vi "ReadSpec校准.vi"() -> (3 "补偿值":T3={"甩线补偿值"={"下边"=23.0, "距离上边"=10.0, "左边"=7.2, "右边"=25.8}, "补偿甩线坐标偏移"={"X"=40.0, "Y"=70.0}, "mark点补偿"={"X"=-48.38, "Y"=-84.85}, "出线补偿值"=25.8, "mark规格"={"X下限"=-48.38, "X上限"=-84.85, "Y下限"=0.0, "Y 上限"=0.0, "angle下限"=0.0, "angle上限"=0.0}} {"mark规格"."angle上限" format="%#.3f"; "mark规格"."angle下限" format="%#.3f"; "mark规格"."Y下限" format="%#.3f"; "mark规格"."X下限" format="%#.3f"; "mark点补偿"."X" format="%#.3f"; "补偿甩线坐标偏移"."X" format="%#.3f"})   [LabVIEW 2014]
uses:
  Controls/XYPos.ctl
  Global.vi
  <vilib>/Utility/file.llb/Read From Spreadsheet File (string).vi
panel:
  out "all rows":string[][](array[string]) caption="所有行"
  out "数组":dbl[](array[numeric])
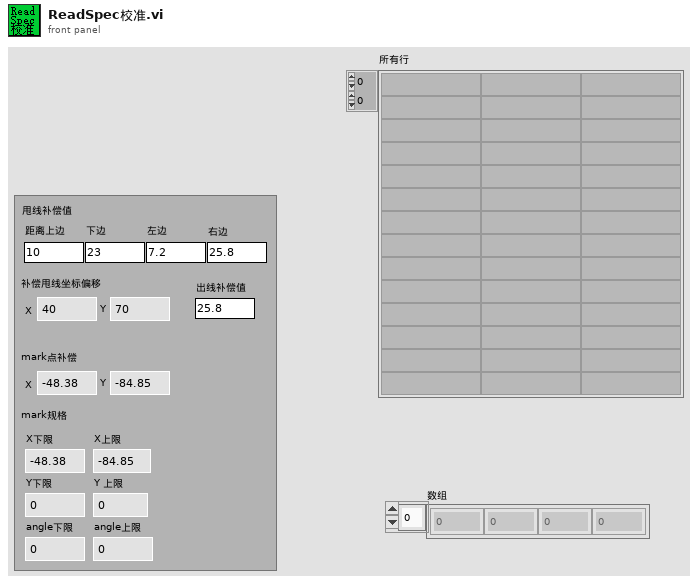
[diagram p1: front panel]
types:
  T1 = typedef "XYPos.ctl" = cluster{"X":dbl, "Y":dbl}
  T2 = typedef "mark规格.ctl" = cluster{"X下限":dbl, "X上限":dbl, "Y下限":dbl, "Y 上限":dbl, "angle下限":dbl, "angle上限":dbl}
  T3 = cluster{"甩线补偿值":cluster{"下边":dbl, "距离上边":dbl, "左边":dbl, "右边":dbl}, "补偿甩线坐标偏移":T1, "mark点补偿":T1, "出线补偿值":dbl, "mark规格":T2}
  T4 = cluster{"[0]":dbl, "[1]":dbl, "[2]":dbl, "[3]":dbl}
  T5 = cluster{"[0]":dbl, "[1]":dbl, "[2]":dbl, "[3]":dbl, "[4]":dbl, "[5]":dbl}
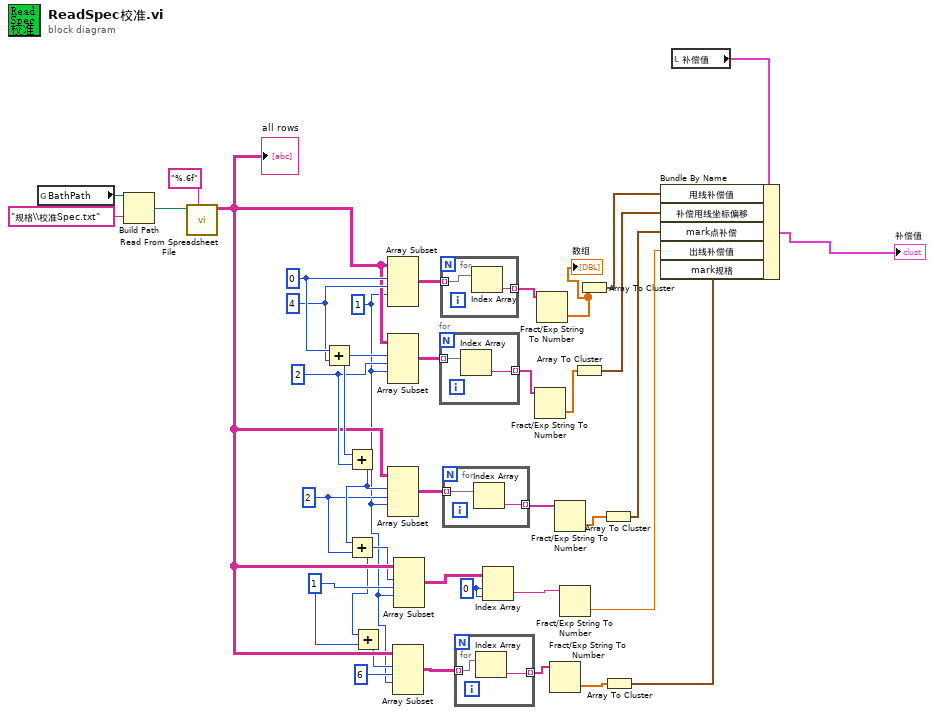
[diagram p0: block diagram]
diagram:
  w11 = 0 ("索引 (行)")
  w9 = 1 ("长度")
  w23 = 2 ("长度")
  w26 = 4
  w18 = 2 ("长度")
  w27 = 0 ("索引")
  w5 = 1 ("索引")
  n1 = global read "Global.vi" "BathPath"() -> (w37:path)
  n2 = Build Path(base path=w37, name or relative path="规格\\校准Spec.txt" ("名称或相对路径")) -> (appended path=w31:path)
  n3 = call-poly <vilib>:"Read From Spreadsheet File.vi"("format (%s)"="%.6f" ("format (%.3f)"), "file path (dialog if empty)"=w31) -> ("all rows"=w10:string[][])  [unwired: 5 in, 4 out]
  "all rows" <- w10
  n4 = Add(x=w27, y=w26) -> (x+y=w24:i32)
  n5 = Add(x=w24, y=w23) -> (x+y=w19:i32)
  n6 = Add(x=w19, y=w18) -> (x+y=w8:i32)
  n7 = Add(x=w8, y=w9) -> (x+y=w7:i32)
  n8 = Array Subset ("数组子集")(array=w10, index (row)=w27, length (row)=w26, index (col)=w5) -> (w35:string[][])  [unwired: 1 in]
  n9 = Array Subset ("数组子集")(array=w10, index (row)=w24, length (row)=w23, index (col)=w5) -> (w33:string[][])  [unwired: 1 in]
  n10 = Array Subset ("数组子集")(array=w10, index (row)=w19, length (row)=w18, index (col)=w5) -> (w30:string[][])  [unwired: 1 in]
  n11 = Array Subset ("数组子集")(array=w10, index (row)=w7, length (row)=6 ("长度"), index (col)=w5) -> (w4:string[][])  [unwired: 1 in]
  n12 = Array Subset ("数组子集")(array=w10, index (row)=w8, length (row)=w9, index (col)=w5) -> (w17:string[][])  [unwired: 1 in]
  n13 = for {
    tunnel: w33 -> [w40] mode=indexing
    tunnel: [w39] -> w22 mode=indexing
    n14 = Index Array(array=w40) -> (element=w39:string)  [unwired: 1 in]
  }
  n15 = for {
    tunnel: w35 -> [w42] mode=indexing
    tunnel: [w41] -> w29 mode=indexing
    n16 = Index Array(array=w42) -> (element=w41:string)  [unwired: 1 in]
  }
  n17 = for {
    tunnel: w30 -> [w44] mode=indexing
    tunnel: [w43] -> w15 mode=indexing
    n18 = Index Array(array=w44) -> (element=w43:string)  [unwired: 1 in]
  }
  n19 = for {
    tunnel: [w46] -> w1 mode=indexing
    tunnel: w4 -> [w45] mode=indexing
    n20 = Index Array(array=w45) -> (element=w46:string)  [unwired: 1 in]
  }
  n21 = Index Array(array=w17, index (row)=w11, index (col)=w11) -> (element=w13:string)
  n22 = Fract/Exp String To Number(string=w22) -> (number=w21:dbl[])  [unwired: 3 in, 1 out]
  n23 = Fract/Exp String To Number(string=w29) -> (number=w28:dbl[])  [unwired: 3 in, 1 out]
  "数组" <- w28
  n24 = Fract/Exp String To Number(string=w1) -> (number=w2:dbl[])  [unwired: 3 in, 1 out]
  n25 = Fract/Exp String To Number(string=w15) -> (number=w14:dbl[])  [unwired: 3 in, 1 out]
  n26 = Fract/Exp String To Number(string=w13) -> (number=w12:dbl)  [unwired: 3 in, 1 out]
  n27 = Array To Cluster(array=w21) -> (cluster=w32:cluster{"[0]":dbl, "[1]":dbl})
  n28 = Array To Cluster(array=w28) -> (cluster=w34:T4)
  n29 = Array To Cluster(array=w14) -> (cluster=w25:cluster{"[0]":dbl, "[1]":dbl})
  n30 = Array To Cluster(array=w2) -> (cluster=w3:T5)
  n31 = local read "补偿值"() -> (w16:T3)
  n32 = Bundle By Name(cluster=w16, "甩线补偿值"=w34, "补偿甩线坐标偏移"=w32, "mark点补偿"=w25, "出线补偿值"=w12, "mark规格"=w3) -> (→"补偿值":T3)
